vi "Rysowanie strzałki kierunkowej.vi"(9 "Lista współrzędnych":string[][](array[string]), 10 "Kierunek na punkt in":u16(ring)) -> (1 "Odległośc do wskazanego punktu poniżej 0,5m":bool, 3 "Mapa ze strzałką":picture)   [LabVIEW 2012]
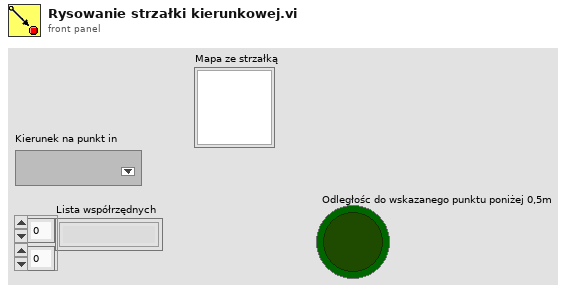
[diagram p1: front panel]
types:
  T1 = cluster{"Położenie grotu":cluster{"Pixel x":i16, "Pixel y":i16}, "Kolor":u32, "Długość [px]":u32, "Kąt/azymut":dbl, "Interpretacją kąta ustawienia strzałki":enum16{"Kąt trygonometryczny", "Azymut"}, "Grubość":u32, "Długość grotu":u32}
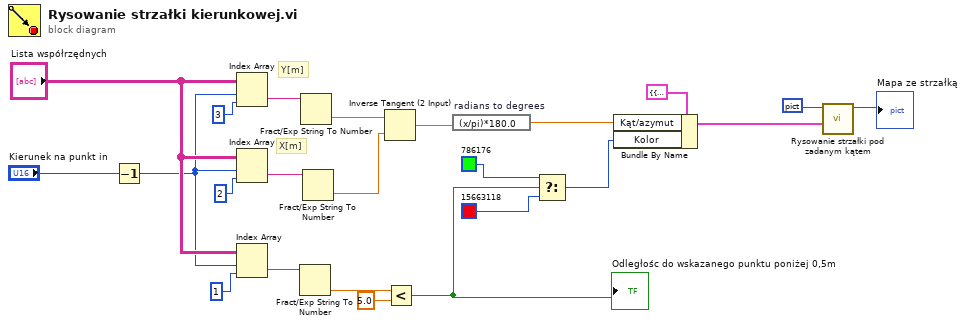
[diagram p0: block diagram]
diagram:
  # "Y[m]"
  # "X[m]"
  n1 = Decrement(x="Kierunek na punkt in") -> (x-1=w9:u16)
  n2 = Index Array(array="Lista współrzędnych", index (row)=w9, index (col)=3 ("disabled index (col)")) -> (element=w17:string)
  n3 = Index Array(array="Lista współrzędnych", index (row)=w9, index (col)=2) -> (element=w16:string)
  n4 = Index Array(array="Lista współrzędnych", index (row)=w9, index (col)=1 ("disabled index (col)")) -> (element=w7:string)
  n5 = Fract/Exp String To Number(string=w7) -> (number=w6:dbl)  [unwired: 3 in, 1 out]
  n6 = Fract/Exp String To Number(string=w17) -> (number=w14:dbl)  [unwired: 3 in, 1 out]
  n7 = Fract/Exp String To Number(string=w16) -> (number=w12:dbl)  [unwired: 3 in, 1 out]
  n8 = Inverse Tangent (2 Input)(1:w12, 2:w14) -> (0:w13:dbl)
  n9 = Less?(x=w6, y=5.0) -> (x < y?=w3:bool)
  "Odległośc do wskazanego punktu poniżej 0,5m" <- w3
  n10 = expression code="(x/pi)*180.0" "radians to degrees"(w13) -> (w11:dbl)
  n11 = Select(t=u32 786176 ("Kolor"), s=w3, f=u32 15663118 ("Kolor")) -> (s? t:f=w2:u32)
  n12 = Bundle By Name(cluster=T1 {"Położenie grotu"={"Pixel x"=100, "Pixel y"=-60}, "Kolor"=0, "Długość [px]"=61, "Kąt/azymut"=200.0, "Interpretacją kąta ustawienia strzałki"=enum."Kąt trygonometryczny", "Grubość"=5, "Długość grotu"=25} ("Parametry strzałki"), "Kąt/azymut"=w11, "Kolor"=w2) -> (w23:T1)
  n13 = call "Rysowanie strzałki pod zadanym kątem.vi"("Parametry strzałki"=w23, "Mapa terenu"=picture data[5B]) -> ("Mapa ze strzałką"=→"Mapa ze strzałką":picture)  [unwired: 9 in]
